vi "Flush Buffer.vi"(8 "error in (no error)":errorcluster, 11 "2D U16 DVR Array in":refnum<class "2D U16 DVR Array.lvclass">) -> (0 "error out":errorcluster, 3 "2D U16 DVR Array out":refnum<class "2D U16 DVR Array.lvclass">)   [LabVIEW 2024, in "2D U16 DVR Array.lvclass"]
uses:
  2D U16 DVR Array.lvclass
  2D U16 DVR Array.lvclass/2D U16 DVR Array.ctl
  Public Data/Write Count.vi
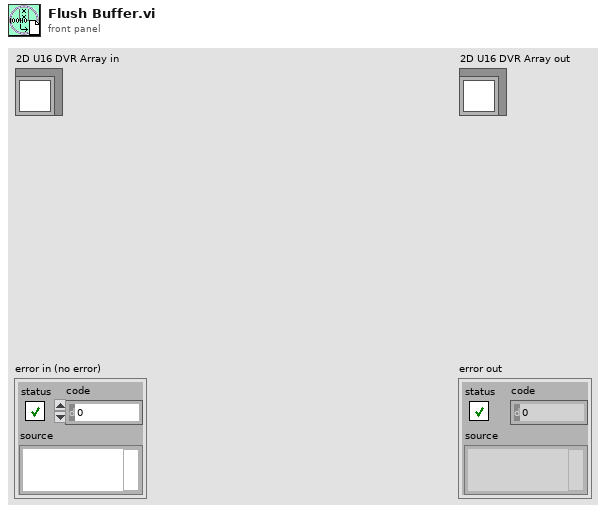
[diagram p1: front panel]
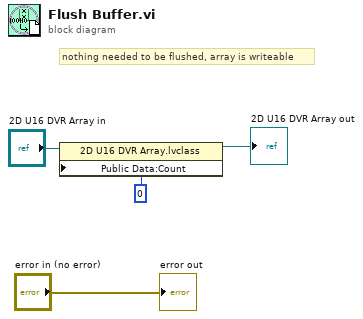
[diagram p0: block diagram]
diagram:
  # "nothing needed to be flushed, array is writeable"
  n1 = property class="2D U16 DVR Array.lvclass"(reference="2D U16 DVR Array in", "Public Data:Count"=0 ("Count")) -> (reference out=→"2D U16 DVR Array out":refnum<class "2D U16 DVR Array.lvclass">)  [unwired: 1 in, 1 out]
  "error out" <- "error in (no error)"
